vi "Configure Modulation (Amplitude).vi"(0 "VISA resource name":refnum<visa-resource-name>, 1 "Enable AM (T:Enable)":bool=TRUE, 2 "AM Path (1)":u16(ring)=1 items=["1"=1, "2"=2, "Wideband"=3], 5 "AM Mode (1: Normal)":u16(ring)=1 items=["Deep", "Normal"], 7 "AM Type (0: Linear)":u16(ring) items=["Linear", "Exponential"], 9 "Enable Depth Coupling (T:Enable)":bool=TRUE, 11 "error in (no error)":errorcluster, 12 "AM Depth (10 percent)":dbl=10.0, 13 "Wideband AM Sensitivity (20 dB)":dbl=20.0) -> (4 "VISA resource name out":refnum<visa-resource-name>, 15 "error out":errorcluster)   [LabVIEW 2011, in "Agilent PSG MXG Series.lvlib"]
doc: "Configures amplitude modulation.\n\n<B>Notes:</B>\n(1) This VI is <B>NOT</B> valid in E8247C.\n\n(2) For E8257D, E8267D, N5181A, N5182A, N5183A, this VI is valid only when the instument installs <B>Option UNT</B> (AM, FM, phase modulation)."
uses:
  Agilent PSG MXG Series.lvlib
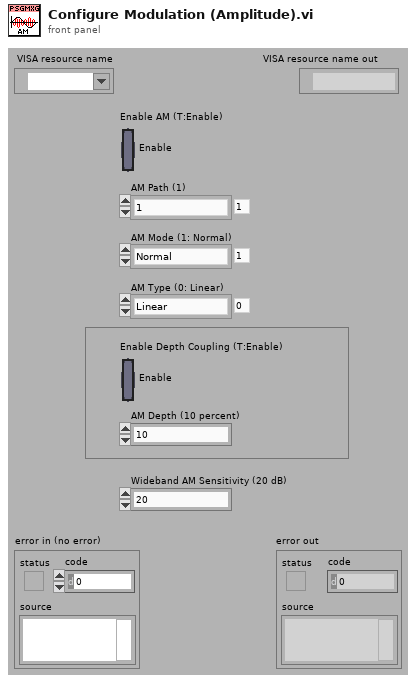
[diagram p1: front panel]
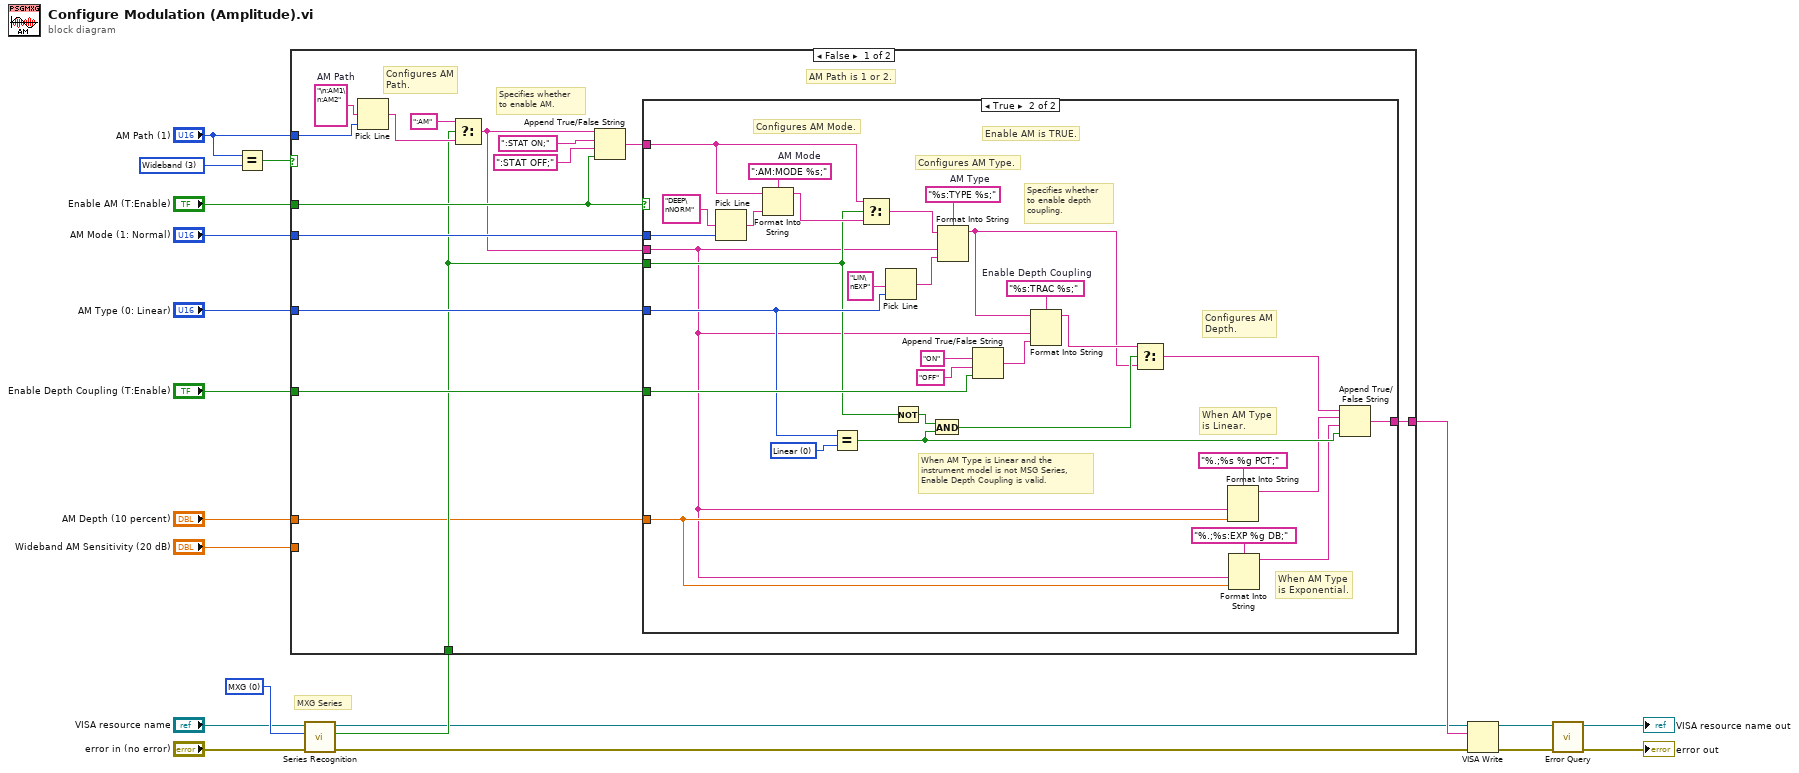
[diagram p0: block diagram]
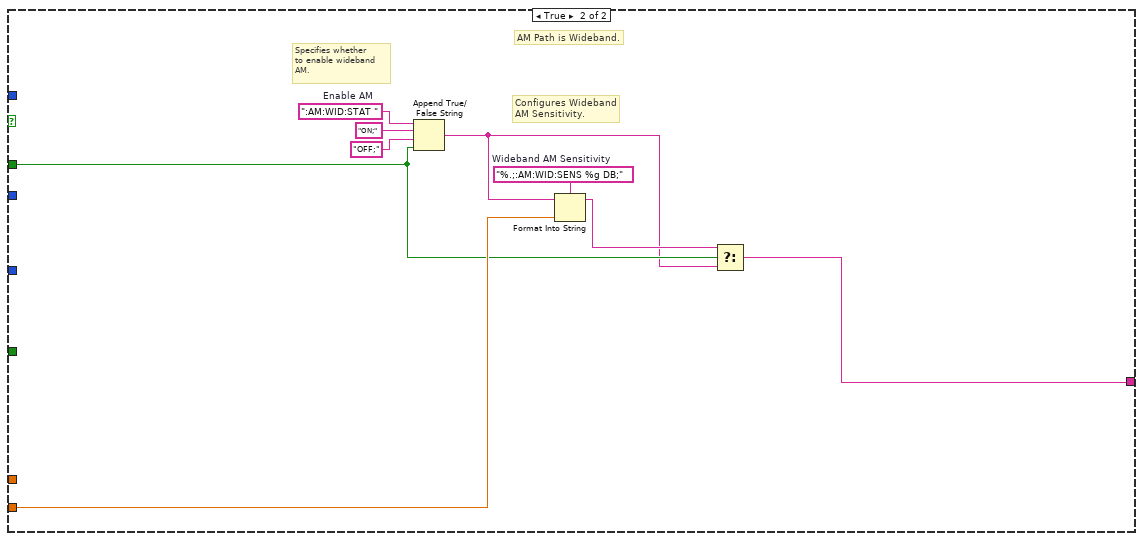
[diagram p3: hidden frame]
diagram:
  w5 = u16 0 items=["MXG", "PSG", "PSG-A", "PSG-C", "PSG-D"] ("Series Type (0: MXG)")
  w20 = u16 3 items=["1"=1, "2"=2, "Wideband"=3] ("AM Path (1)")
  # "MXG Series"
  n1 = Equal?(x="AM Path (1)", y=w20) -> (x = y?=w19:bool)
  n2 = call "Series Recognition.vi"("error in (no error)"="error in (no error)", "Series Type (0: MXG)"=w5, "VISA resource name"="VISA resource name") -> ("error out"=w7:errorcluster, "Is Series Correct"=w8:bool, "VISA resource name out"=w6:refnum<visa-resource-name>)  [unwired: 6 in]
  n3 = case shown="False" w19 {
    tunnel: "AM Path (1)" -> [w34 _]
    tunnel: "Enable AM (T:Enable)" -> [w28 w71]
    tunnel: "AM Mode (1: Normal)" -> [w31 _]
    tunnel: w8 -> [w25 _]
    tunnel: "AM Type (0: Linear)" -> [w27 _]
    tunnel: "Enable Depth Coupling (T:Enable)" -> [w26 _]
    tunnel: "AM Depth (10 percent)" -> [w23 _]
    tunnel: [w22 w68] -> w12
    tunnel: "Wideband AM Sensitivity (20 dB)" -> [_ w72]
    frame False {
      w35 = "\n:AM1\n:AM2"  # AM Path
      # "Specifies whether\nto enable AM."
      # "Configures AM\nPath."
      # "AM Path is 1 or 2."
      n4 = Pick Line(multi-line string=w35, line index=w34) -> (output string=w30:string)  [unwired: 1 in]
      n5 = Select(t=":AM", s=w25, f=w30) -> (s? t:f=w24:string)
      n6 = Append True/False String(1:w28, 2:":STAT OFF;" ("false string"), 3:":STAT ON;" ("true string"), 4:w24) -> (0:w32:string)
      n7 = case shown="True" w28 {
        tunnel: w32 -> [w36 w63]
        tunnel: w31 -> [_ w64]
        tunnel: w25 -> [_ w49]
        tunnel: w27 -> [_ w52]
        tunnel: w24 -> [_ w37]
        tunnel: w26 -> [_ w53]
        tunnel: w23 -> [_ w43]
        tunnel: [w36 w38] -> w22
        frame False {
          # "Enable AM is FALSE."
        }
        frame True {
          w51 = u16 0 items=["Linear", "Exponential"] ("AM Type (0: Linear)")
          w57 = "%s:TRAC %s;"  # Enable Depth Coupling
          w60 = "%s:TYPE %s;"  # AM Type
          w67 = ":AM:MODE %s;"  # AM Mode
          # "When AM Type\nis Exponential."
          # "When AM Type\nis Linear."
          # "Configures AM\nDepth."
          # "When AM Type is Linear and the\ninstrument model is not MSG Series,\nEnable Depth Coupling is valid."
          # "Specifies whether\nto enable depth\ncoupling."
          # "Configures AM Type."
          # "Configures AM Mode."
          # "Enable AM is TRUE."
          n8 = Pick Line(multi-line string="DEEP\nNORM", line index=w64) -> (output string=w66:string)  [unwired: 1 in]
          n9 = Format Into String(format string=w67, initial string=w63, w66) -> (resulting string=w62:string)  [unwired: 1 in, 1 out]
          n10 = Equal?(x=w52, y=w51) -> (x = y?=w42:bool)
          n11 = Select(t=w63, s=w49, f=w62) -> (s? t:f=w61:string)
          n12 = Pick Line(multi-line string="LIN\nEXP", line index=w52) -> (output string=w58:string)  [unwired: 1 in]
          n13 = Not(x=w49) -> (.not. x?=w50:bool)
          n14 = And(x=w50, y=w42) -> (x .and. y?=w48:bool)
          n15 = Format Into String(format string=w60, initial string=w61, w37, w58) -> (resulting string=w46:string)  [unwired: 1 in, 1 out]
          n16 = Append True/False String(1:w53, 2:"OFF" ("false string"), 3:"ON" ("true string")) -> (0:w56:string)  [unwired: 1 in]
          n17 = Format Into String(format string=w57, initial string=w46, w37, w56) -> (resulting string=w47:string)  [unwired: 1 in, 1 out]
          n18 = Select(t=w47, s=w48, f=w46) -> (s? t:f=w39:string)
          n19 = Format Into String(format string="%.;%s %g PCT;", w37, w43) -> (resulting string=w41:string)  [unwired: 2 in, 1 out]
          n20 = Format Into String(format string="%.;%s:EXP %g DB;", w37, w43) -> (resulting string=w40:string)  [unwired: 2 in, 1 out]
          n21 = Append True/False String(1:w42, 2:w40, 3:w41, 4:w39) -> (0:w38:string)
        }
      }
    }
    frame True {
      w73 = "%.;:AM:WID:SENS %g DB;"  # Wideband AM Sensitivity
      w76 = ":AM:WID:STAT "  # Enable AM
      # "Configures Wideband\nAM Sensitivity."
      # "Specifies whether\nto enable wideband\nAM."
      # "AM Path is Wideband."
      n22 = Append True/False String(1:w71, 2:"OFF;" ("false string"), 3:"ON;" ("true string"), 4:w76) -> (0:w69:string)
      n23 = Format Into String(format string=w73, initial string=w69, w72) -> (resulting string=w70:string)  [unwired: 1 in, 1 out]
      n24 = Select(t=w70, s=w71, f=w69) -> (s? t:f=w68:string)
    }
  }
  n25 = VISA Write(VISA resource name=w6, write buffer=w12, error in (no error)=w7) -> (VISA resource name out=w11:refnum<visa-resource-name>, error out=w10:errorcluster)  [unwired: 1 out]
  n26 = call "Error Query.vi"("error in (no error)"=w10, "VISA resource name"=w11) -> ("error out"=→"error out":errorcluster, "VISA resource name out"=→"VISA resource name out":refnum<visa-resource-name>)  [unwired: 6 in, 2 out]
